vi "FilterSwitcher.vi"(8 "error in (no error)":errorcluster, 9 "Filter Change Speed":i32, 10 "Filter Position":i32=6) -> (0 "error out":errorcluster)   [LabVIEW 2015]
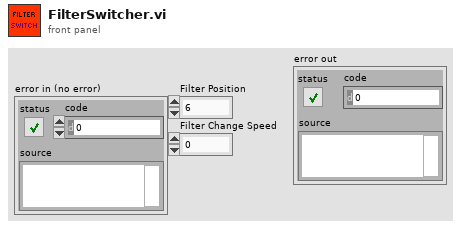
[diagram p1: front panel]
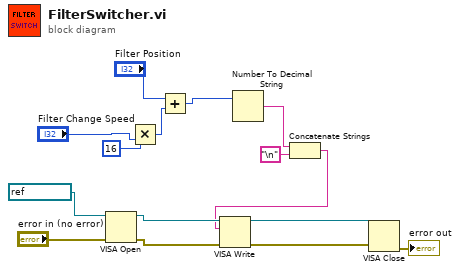
[diagram p0: block diagram]
diagram:
  n1 = VISA Open(error in (no error)="error in (no error)", VISA resource name=refnum<visa-resource-name> "COM14") -> (VISA resource name=w14:refnum<visa-resource-name>, error out=w13:errorcluster)  [unwired: 3 in]
  n2 = Multiply(x=16, y="Filter Change Speed") -> (x*y=w6:i32)
  n3 = Add(x="Filter Position", y=w6) -> (x+y=w5:i32)
  n4 = Number To Decimal String(number=w5) -> (decimal integer string=w4:string)  [unwired: 1 in]
  n5 = Concatenate Strings(w4, "\n" ("string")) -> (w3:string)
  n6 = VISA Write(VISA resource name=w14, write buffer=w3, error in (no error)=w13) -> (VISA resource name out=w10:refnum<visa-resource-name>, error out=w11:errorcluster)  [unwired: 1 out]
  n7 = VISA Close(VISA resource name=w10, error in (no error)=w11) -> (error out=→"error out":errorcluster)
